vi "hse-application_VersionNumber--constant.vi"() -> (3 "HSE-Libraries Version Number":string="dev. env.")   [LabVIEW 2014, in "hse-application.lvclass"]
uses:
  hse-application.lvclass
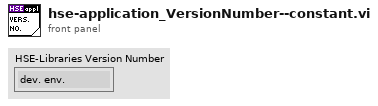
[diagram p1: front panel]
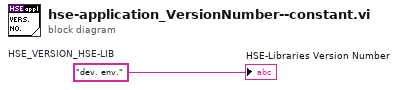
[diagram p0: block diagram]
diagram:
  w1 = "dev. env."  # HSE_VERSION_HSE-LIB
  "HSE-Libraries Version Number" <- w1
